vi "for.vi"() -> ()   [LabVIEW 2020]
panel:
  out "x*y":dbl
  out "Numeric":i32
  in  "Numeric 2":i32
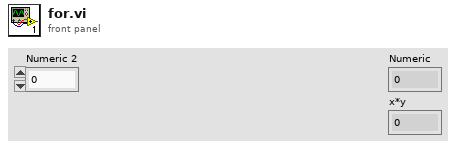
[diagram p1: front panel]
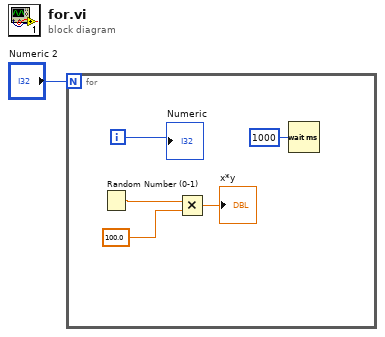
[diagram p0: block diagram]
diagram:
  n1 = for {
    N: "Numeric 2" -> [_]
    i -> [w6]
    n2 = Random Number (0-1)() -> (number: 0 to 1=w3:dbl)
    n3 = Multiply(x=w3, y=100.0) -> (x*y=→"x*y":dbl)
    n4 = Wait (ms)(milliseconds to wait=u32 1000) -> ()  [unwired: 1 out]
    "Numeric" <- w6
  }
